vi "ClientProcess.vi"(0 "occurrence":refnum<k4>, 1 "target address":string, 2 "TCP port":u16, 5 "error in (no error)":errorcluster) -> (19 "error out":errorcluster)   [LabVIEW 2017, in "G#RemoteProxy.lvclass"]
doc: "Client process for the remote link to the target server process."
uses:
  G#RemoteProxy.lvclass
  G#Object/utils/G#Object_Event.ctl
  G#Object/utils/G#Object_EventType.ctl
  G#Object/utils/G#Object_ObjectInfoType.ctl
  G#Object/utils/G#Object_CreateMethod.ctl
  G#Object/G#Object.lvclass
  G#DebugServer/utils/LocalProcessData.ctl
  G#DebugServer/utils/TCPCommand.ctl
  G#Object/utils/G#Object_ClassInfoType.ctl
  G#Object/utils/G#Object_ClassHierarchy.ctl
  G#Debugger.lvlib
  G#DebugServer/G#DebugServer.lvclass
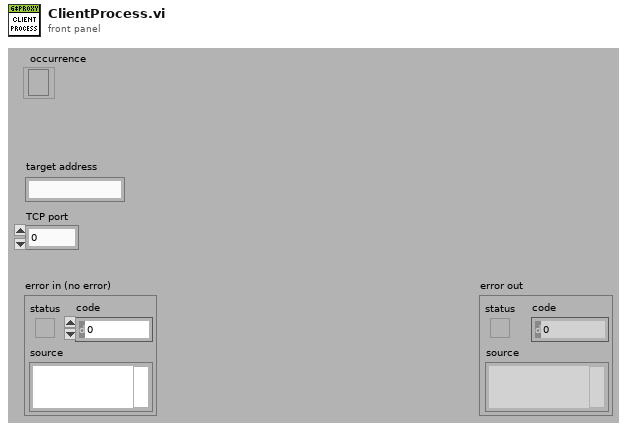
[diagram p1: front panel]
types:
  T1 = cluster{"connection ID":refnum<k5>, "Connected":bool}
  T2 = cluster{"connection ID":refnum<k5>, "Address":u32}
  T3 = typedef "G#Object.lvclass/G#Object_ClassInfoType.ctl" = cluster{"ClassName":string, "ObjectInfo":T4[], "ObjectRefs":refnum<class "G#Object.lvclass">[], "TypeRef":refnum<class "G#Object.lvclass">}
  T4 = typedef "G#Object.lvclass/G#Object_ObjectInfoType.ctl" = cluster{"ObjectName":string, "ObjectID":u32, "Users":i32, "Counter":bool, "AttributeRefs":u32[], "FullClassName":string, "ClassName":string, "CreateMethod":T5, "GenericDestructorExists":bool, "Owner":string}
  T5 = typedef "G#Object.lvclass/G#Object_CreateMethod.ctl" = enum16{"Create", "Create or look up existing", "Look up existing"}
  T6 = typedef "G#Object.lvclass/G#Object_ClassHierarchy.ctl" = cluster{"ClassName":string, "FullClassName":string, "ClassPath":path, "IsLeaf":bool}
  T7 = cluster{"AllObjects":T3, "class hierarchy":T6[]}[]
  T8 = typedef "G#DebugServer.lvclass/LocalProcessData.ctl" = cluster{"Event":string, "Command":T9, "Data":string, "Address":u32}
  T9 = typedef "G#DebugServer.lvclass/TCPCommand.ctl" = u8
  T10 = typedef "G#Object.lvclass/G#Object_Event.ctl" = cluster{"EventType":T11, "ObjectInfo":T4, "Ref":refnum<class "G#Object.lvclass">, "Time Stamp":timestamp, "LogText":string, "Parameters":variant[]}
  T11 = typedef "G#Object.lvclass/G#Object_EventType.ctl" = enum16{"Created new", "Looked up existing", "Deleted", "Forced delete", "Not deleted", "Garbage collected", "Cleared", "User", "Error", "External create object", "External create class attributes", "Created class attributes", "Run constructor", "Run constructor done", "Run open method", "Run open method done"}
  T12 = cluster{"G#DebugServerRef":refnum<class "G#Object.lvclass">, "attributes":variant[]}
  T13 = cluster{"G#DebugServerRef":refnum<class "G#Object.lvclass">, "ToString":string}
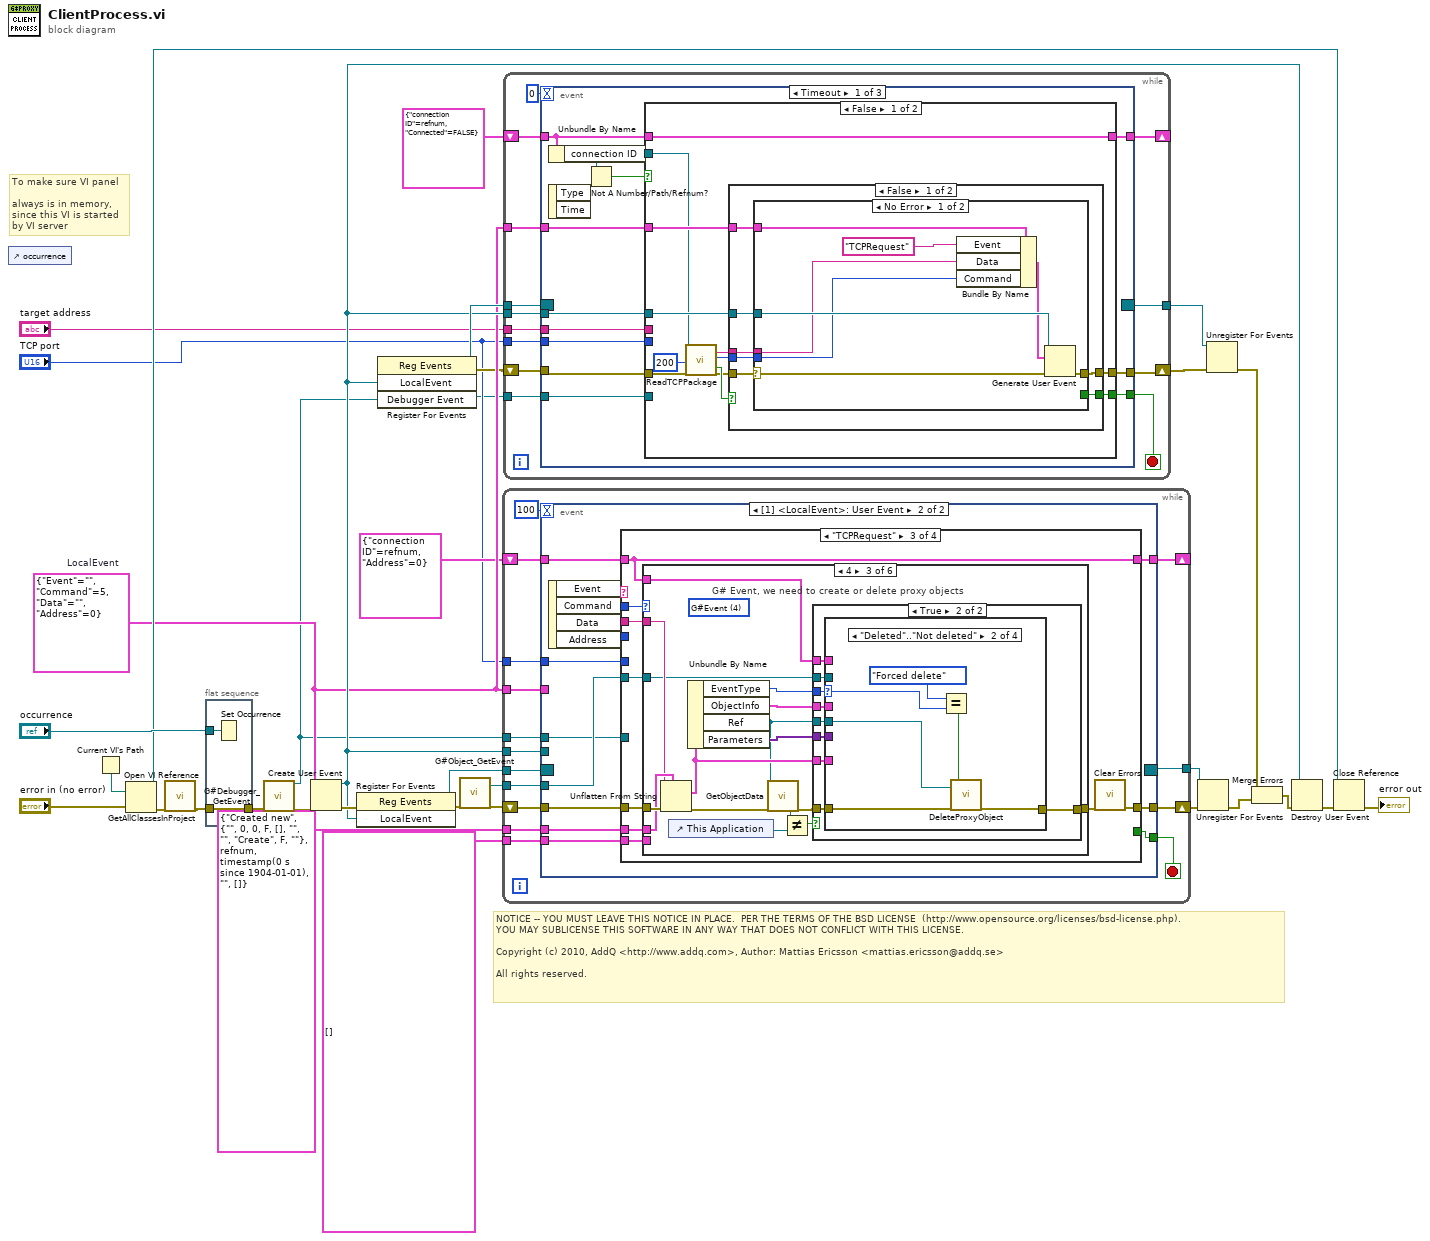
[diagram p0: block diagram]
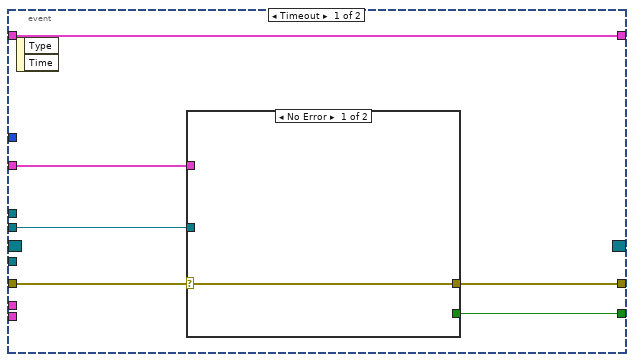
[diagram p2: hidden frame]
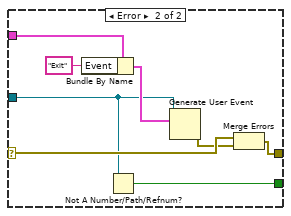
[diagram p3: hidden frame]
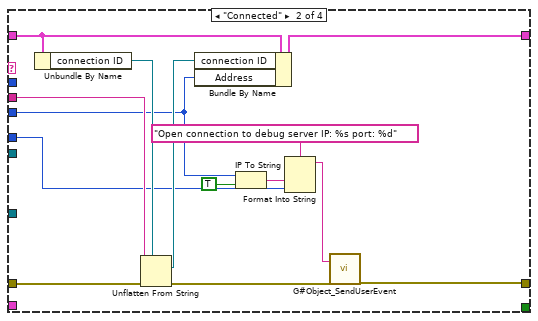
[diagram p5: hidden frame]
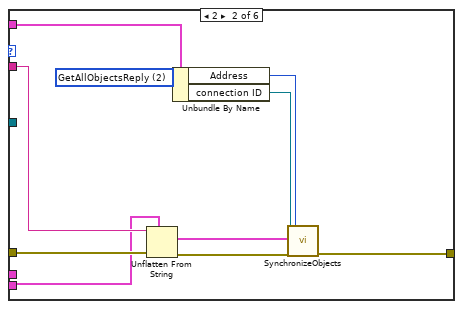
[diagram p7: hidden frame]
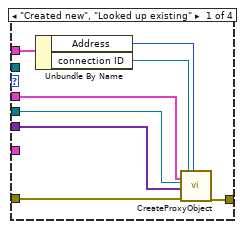
[diagram p9: hidden frame]
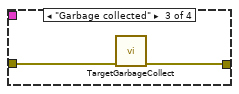
[diagram p10: hidden frame]
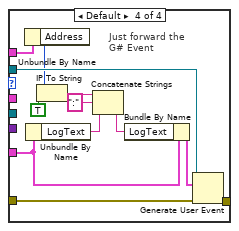
[diagram p11: hidden frame]
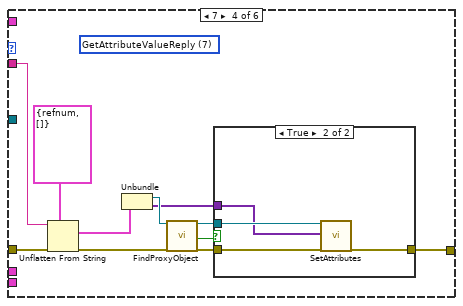
[diagram p12: hidden frame]
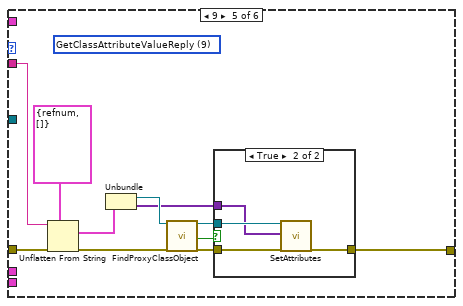
[diagram p14: hidden frame]
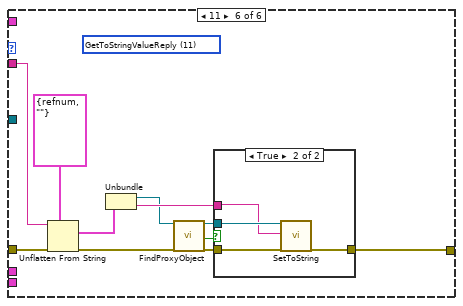
[diagram p16: hidden frame]
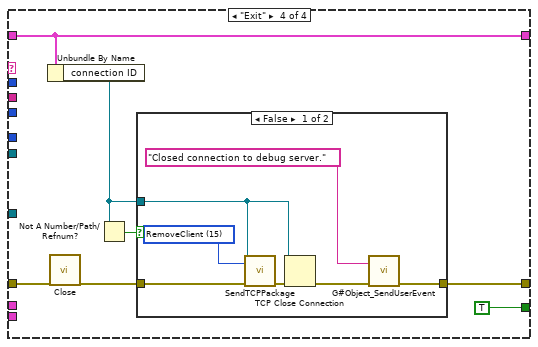
[diagram p18: hidden frame]
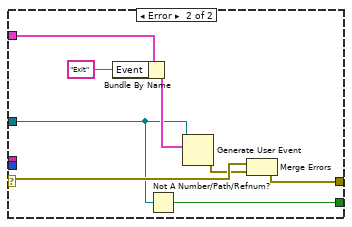
[diagram p20: hidden frame]
diagram:
  w12 = T8 {"Event"="", "Command"=5, "Data"="", "Address"=0}  # LocalEvent
  # "NOTICE -- YOU MUST LEAVE THIS NOTICE IN PLACE.  PER THE TERMS OF THE BSD LICENSE  (http://www.opensource.org/licenses/bsd-license.php).\nYOU MAY SUBLICENSE THIS SOFTWARE IN ANY WAY THAT DOES NOT CONFLICT WITH THIS LICENSE.\n\nCopyright (c) 2010, AddQ <http://www.addq.com>, Author: Mattias Ericsson <mattias.ericsson@addq.se>\n\nAll rights reserved."
  # "To make sure VI panel\n\nalways is in memory,\nsince this VI is started\nby VI server"
  n1 = control-ref of="occurrence"() -> ()  [unwired: 1 out]
  n2 = Current VI's Path() -> (path=w33:path)
  n3 = Open VI Reference(vi path=w33, error in (no error)="error in (no error)") -> (vi reference=w29:refnum<vi>, error out=w10:errorcluster)  [unwired: 4 in]
  n4 = call "GetAllClassesInProject.vi"("error in (no error)"=w10) -> ("error out"=w6:errorcluster)  [unwired: 15 in, 3 out]
  n5 = flat-sequence {
    tunnel: "occurrence" -> [w35]
    tunnel: w6 -> [w34]
    tunnel: [w34] -> w9
    frame #0 {
      n6 = Set Occurrence(w35) -> ()
    }
  }
  n7 = call "G#Debugger_GetEvent.vi"("error in (no error)"=w9) -> ("Debugger Event"=w2:refnum<user-event>, "error out"=w28:errorcluster)  [unwired: 17 in]
  n8 = Create User Event(user event datatype=w12, error in=w28) -> (user event=w13:refnum<user-event>, error out=w27:errorcluster)
  n9 = register-events(error in=w27, w13) -> (reference out=w19:refnum<event-registration>, error out=w26:errorcluster)  [unwired: 1 in]
  n10 = register-events(w13, w2) -> (reference out=w24:refnum<event-registration>, error out=w4:errorcluster)  [unwired: 2 in]
  n11 = call "G#Object_GetEvent.vi"("error in (no error)"=w26) -> ("G# event"=w15:refnum<user-event>, "error out"=w25:errorcluster)  [unwired: 14 in, 3 out]
  n12 = while {
    shift-right: [w46] -> w21
    shift-left: w25 -> [w49]
    tunnel: [w50] -> w20
    tunnel: w19 -> [w48]
    tunnel: w13 -> [w45]
    tunnel: w15 -> [w43]
    tunnel: T10 {"EventType"=enum."Created new", "ObjectInfo"={"ObjectName"="", "ObjectID"=0, "Users"=0, "Counter"=FALSE, "AttributeRefs"=[], "FullClassName"="", "ClassName"="", "CreateMethod"=enum."Create", "GenericDestructorExists"=FALSE, "Owner"=""}, "Ref"=refnum, "Time Stamp"=timestamp(0 s since 1904-01-01), "LogText"="", "Parameters"=[]} ("event data") -> [w42]
    tunnel: w12 -> [w41]
    tunnel: T7 [] ("TargetClassInfo") -> [w40]
    shift-right: [w38] -> _
    shift-left: T2 {"connection ID"=refnum, "Address"=0} -> [w39]
    tunnel: "TCP port" -> [w37]
    tunnel: w2 -> [w36]
    stop <- w44 stop-if-true
    n13 = event shown="[1] <LocalEvent>: User Event" {
      selector: w48 -> [_ _]
      dyn-events: [_ _] -> w50
      timeout: 100 -> [_ _]
      tunnel: w49 -> [w56 w78]
      tunnel: [w54 w77] -> w46
      tunnel: w45 -> [w55 _]
      tunnel: [w52 w76] -> w44
      tunnel: w43 -> [_ w73]
      tunnel: w42 -> [_ w72]
      tunnel: w41 -> [w53 _]
      tunnel: w40 -> [_ w71]
      tunnel: w39 -> [w51 w70]
      tunnel: [w51 w69] -> w38
      tunnel: w37 -> [_ w67]
      tunnel: w36 -> [_ w66]
      event Timeout {
        n14 = event-data() -> ()  [unwired: 1 in, 2 out]
        n15 = case shown="No Error" w56 {
          selector: w56 -> [w57 w64]
          tunnel: w55 -> [_ w59]
          tunnel: [w57 w65] -> w54
          tunnel: w53 -> [_ w62]
          tunnel: [_ w58] -> w52
          frame No Error {
          }
          frame Error {
            n16 = Bundle By Name(cluster=w62, "Event"="Exit") -> (w61:T8)
            n17 = Not A Number/Path/Refnum?(number/path/refnum=w59) -> (NaN/Path/Refnum?=w58:bool)
            n18 = Generate User Event(user event=w59, event data cluster=w61) -> (error out=w63:errorcluster)  [unwired: 2 in, 1 out]
            n19 = Merge Errors(w64, w63) -> (w65:errorcluster)
          }
        }
      }
      event User Event {
        n20 = event-data() -> ("Event"=w79:string, "Command"=w75:T9, "Data"=w74:string, "Address"=w68:u32)  [unwired: 1 in]
        n21 = case shown="\"TCPRequest\"" w79 {
          tunnel: w78 -> [w81 w95 w101 w222]
          tunnel: [w81 w82 w97 w219] -> w77
          tunnel: [_ _ _ TRUE] -> w76
          tunnel: w75 -> [_ _ w104 _]
          tunnel: w74 -> [_ w94 w103 _]
          tunnel: w73 -> [_ _ w102 _]
          tunnel: w72 -> [_ _ w100 _]
          tunnel: w71 -> [_ _ w99 _]
          tunnel: w70 -> [w80 w92 w96 w218]
          tunnel: [w80 w91 w96 w218] -> w69
          tunnel: w68 -> [_ w85 _ _]
          tunnel: w67 -> [_ w83 _ _]
          tunnel: w66 -> [_ _ _ _]
          frame Default {
          }
          frame "Connected" {
            n22 = Unbundle By Name(w92) -> ("connection ID"=w93:refnum<k5>)
            n23 = Unflatten From String(type=w93, binary string=w94, error in (no error)=w95) -> (value=w90:refnum<k5>, error out=w89:errorcluster)  [unwired: 2 in, 1 out]
            n24 = Bundle By Name(cluster=w92, "connection ID"=w90, "Address"=w85) -> (w91:T2)
            n25 = IP To String(1:TRUE ("dot notation? (F)"), 2:w85) -> (0:w86:string)
            n26 = Format Into String(format string="Open connection to debug server IP: %s port: %d", w86, w83) -> (resulting string=w87:string)  [unwired: 2 in, 1 out]
            n27 = call "G#Object_SendUserEvent.vi"("text"=w87, "error in (no error)"=w89) -> ("error out"=w82:errorcluster)  [unwired: 16 in, 1 out]
          }
          frame "TCPRequest" {
            n28 = case shown="4" w104 {
              tunnel: w103 -> [_ w113 w128 w178 w194 w210]
              tunnel: w102 -> [_ _ w124 _ _ _]
              tunnel: w101 -> [w105 w114 w130 w179 w195 w211]
              tunnel: [w105 w109 w126 w175 w185 w206] -> w98
              tunnel: w100 -> [_ _ w129 _ _ _]
              tunnel: w99 -> [_ w112 _ _ _ _]
              tunnel: w96 -> [_ w108 w115 _ _ _]
              frame Default {
              }
              frame 2 {
                (unwired) T9 2 items=["GarbageCollect", "GetAllObjects", "GetAllObjectsReply", "CleanUp", "G#Event"] ("Command")
                n29 = Unflatten From String(type=w112, binary string=w113, error in (no error)=w114) -> (value=w110:T7, error out=w111:errorcluster)  [unwired: 2 in, 1 out]
                n30 = Unbundle By Name(w108) -> ("Address"=w107:u32, "connection ID"=w106:refnum<k5>)
                n31 = call "SynchronizeObjects.vi"("connection ID"=w106, "TargetClassInfo"=w110, "error in (no error)"=w111, "address"=w107) -> ("error out"=w109:errorcluster)  [unwired: 15 in]
              }
              frame 4 {
                (unwired) T9 4 items=["GarbageCollect", "GetAllObjects", "GetAllObjectsReply", "CleanUp", "G#Event"] ("Command")
                # "G# Event, we need to create or delete proxy objects"
                n32 = Unflatten From String(type=w129, binary string=w128, error in (no error)=w130) -> (value=w123:T10, error out=w120:errorcluster)  [unwired: 2 in, 1 out]
                n33 = control-ref of="This Application"() -> (w116:refnum<vi>)
                n34 = Unbundle By Name(w123) -> ("EventType"=w127:T11, "ObjectInfo"=w125:T4, "Ref"=w119:refnum<class "G#Object.lvclass">, "Parameters"=w122:variant[])
                n35 = call "GetObjectData.vi"("remote ref"=w119, "error in (no error)"=w120) -> ("AppRefnum"=w117:refnum<vi>, "error out"=w121:errorcluster)  [unwired: 13 in, 3 out]
                n36 = Not Equal?(x=w117, y=w116) -> (x != y?=w118:bool)
                n37 = case shown="True" w118 {
                  tunnel: w127 -> [_ w140]
                  tunnel: w121 -> [w131 w139]
                  tunnel: [w131 w138] -> w126
                  tunnel: w125 -> [_ w137]
                  tunnel: w119 -> [_ w136]
                  tunnel: w124 -> [_ w135]
                  tunnel: w123 -> [_ w134]
                  tunnel: w122 -> [_ w133]
                  tunnel: w115 -> [_ w132]
                  frame False {
                    # "Debug server is running on the\nsame application instance as the debugger,\nthe debugger will catch the event by him self!"
                  }
                  frame True {
                    n38 = case shown="\"Deleted\"..\"Not deleted\"" w140 {
                      selector: w140 -> [_ w151 _ _]
                      tunnel: w139 -> [w148 w154 w156 w168]
                      tunnel: [w147 w153 w155 w167] -> w138
                      tunnel: w137 -> [w144 _ _ _]
                      tunnel: w136 -> [w146 w152 _ _]
                      tunnel: w135 -> [_ _ _ w166]
                      tunnel: w134 -> [_ _ _ w165]
                      tunnel: w133 -> [w145 _ _ _]
                      tunnel: w132 -> [w143 _ _ w160]
                      frame "Created new", "Looked up existing" {
                        n39 = Unbundle By Name(w143) -> ("Address"=w142:u32, "connection ID"=w141:refnum<k5>)
                        n40 = call "CreateProxyObject.vi"("object info"=w144, "remote object ref"=w146, "parameters"=w145, "error in (no error)"=w148, "connection ID"=w141, "address"=w142) -> ("error out"=w147:errorcluster)  [unwired: 13 in]
                      }
                      frame "Deleted".."Not deleted" {
                        n41 = Equal?(x=G#Object_EventType."Forced delete" ("EventType"), y=w151) -> (x = y?=w149:bool)
                        n42 = call "DeleteProxyObject.vi"("remote object ref"=w152, "error in (no error)"=w154, "force delete? (F)"=w149) -> ("error out"=w153:errorcluster)  [unwired: 16 in]
                      }
                      frame "Garbage collected" {
                        n43 = call "TargetGarbageCollect.vi"("error in (no error)"=w156) -> ("error out"=w155:errorcluster)  [unwired: 18 in]
                      }
                      frame Default {
                        # "Just forward the\nG# Event"
                        n44 = Unbundle By Name(w160) -> ("Address"=w158:u32)
                        n45 = Unbundle By Name(w165) -> ("LogText"=w163:string)
                        n46 = IP To String(1:TRUE ("dot notation? (F)"), 2:w158) -> (0:w159:string)
                        n47 = Concatenate Strings(w159, ":" ("string"), w163) -> (w162:string)
                        n48 = Bundle By Name(cluster=w165, "LogText"=w162) -> (w164:T10)
                        n49 = Generate User Event(user event=w166, event data cluster=w164, error in=w168) -> (error out=w167:errorcluster)  [unwired: 1 in, 1 out]
                      }
                    }
                  }
                }
              }
              frame 7 {
                (unwired) T9 7 items=["GarbageCollect", "GetAllObjects", "GetAllObjectsReply", "CleanUp", "G#Event", "RegisterClient", "GetAttributeValue", "GetAttributeValueReply", "GetClassAttributeValue", "GetClassAttributeValueReply", "GetToStringValue", "GetToStringValueReply", "GetClassHierarchy", "GetClassHierarchyReply"] ("Command")
                n50 = Unflatten From String(type=T12 {"G#DebugServerRef"=refnum, "attributes"=[]} ("cluster"), binary string=w178, error in (no error)=w179) -> (value=w176:T12, error out=w174:errorcluster)  [unwired: 2 in, 1 out]
                n51 = Unbundle(w176) -> ("G#DebugServerRef"=w172:refnum<class "G#Object.lvclass">, "attributes"=w169:variant[])
                n52 = call "FindProxyObject.vi"("remote ref"=w172, "error in (no error)"=w174) -> ("proxy ref"=w171:refnum<class "G#RemoteProxy.lvclass">, "found"=w170:bool, "error out"=w173:errorcluster)  [unwired: 15 in]
                n53 = case shown="True" w170 {
                  tunnel: w173 -> [w180 w182]
                  tunnel: [w180 w184] -> w175
                  tunnel: w171 -> [_ w183]
                  tunnel: w169 -> [_ w181]
                  frame False {
                  }
                  frame True {
                    n54 = call "SetAttributes.vi"("reference in"=w183, "attributes"=w181, "error in (no error)"=w182) -> ("error out"=w184:errorcluster)  [unwired: 15 in, 1 out]
                  }
                }
              }
              frame 9 {
                (unwired) T9 9 items=["GarbageCollect", "GetAllObjects", "GetAllObjectsReply", "CleanUp", "G#Event", "RegisterClient", "GetAttributeValue", "GetAttributeValueReply", "GetClassAttributeValue", "GetClassAttributeValueReply", "GetToStringValue", "GetToStringValueReply", "GetClassHierarchy", "GetClassHierarchyReply"] ("Command")
                n55 = Unflatten From String(type=T12 {"G#DebugServerRef"=refnum, "attributes"=[]} ("cluster"), binary string=w194, error in (no error)=w195) -> (value=w192:T12, error out=w191:errorcluster)  [unwired: 2 in, 1 out]
                n56 = Unbundle(w192) -> ("G#DebugServerRef"=w189:refnum<class "G#Object.lvclass">, "attributes"=w186:variant[])
                n57 = call "FindProxyClassObject.vi"("remote class ref"=w189, "error in (no error)"=w191) -> ("proxy class ref"=w188:refnum<class "G#RemoteProxy.lvclass">, "found"=w187:bool, "error out"=w190:errorcluster)  [unwired: 15 in]
                n58 = case shown="True" w187 {
                  tunnel: w190 -> [w196 w200]
                  tunnel: [w196 w199] -> w185
                  tunnel: w188 -> [_ w198]
                  tunnel: w186 -> [_ w197]
                  frame False {
                  }
                  frame True {
                    n59 = call "SetAttributes.vi"("reference in"=w198, "attributes"=w197, "error in (no error)"=w200) -> ("error out"=w199:errorcluster)  [unwired: 15 in, 1 out]
                  }
                }
              }
              frame 11 {
                (unwired) T9 11 items=["GarbageCollect", "GetAllObjects", "GetAllObjectsReply", "CleanUp", "G#Event", "RegisterClient", "GetAttributeValue", "GetAttributeValueReply", "GetClassAttributeValue", "GetClassAttributeValueReply", "GetToStringValue", "GetToStringValueReply", "GetClassHierarchy", "GetClassHierarchyReply"] ("Command")
                n60 = Unflatten From String(type=T13 {"G#DebugServerRef"=refnum, "ToString"=""} ("cluster"), binary string=w210, error in (no error)=w211) -> (value=w208:T13, error out=w205:errorcluster)  [unwired: 2 in, 1 out]
                n61 = Unbundle(w208) -> ("G#DebugServerRef"=w201:refnum<class "G#Object.lvclass">, "ToString"=w207:string)
                n62 = call "FindProxyObject.vi"("remote ref"=w201, "error in (no error)"=w205) -> ("proxy ref"=w202:refnum<class "G#RemoteProxy.lvclass">, "found"=w203:bool, "error out"=w204:errorcluster)  [unwired: 15 in]
                n63 = case shown="True" w203 {
                  tunnel: w204 -> [w212 w216]
                  tunnel: [w212 w215] -> w206
                  tunnel: w202 -> [_ w214]
                  tunnel: w207 -> [_ w213]
                  frame False {
                  }
                  frame True {
                    n64 = call "SetToString.vi"("reference in"=w214, "to string"=w213, "error in (no error)"=w216) -> ("error out"=w215:errorcluster)  [unwired: 15 in, 1 out]
                  }
                }
              }
            }
            n65 = call <vilib>:"Clear Errors.vi"("error in (no error)"=w98) -> ("error out"=w97:errorcluster)  [unwired: 5 in, 1 out]
          }
          frame "Exit" {
            n66 = Unbundle By Name(w218) -> ("connection ID"=w217:refnum<k5>)
            n67 = call "Close.vi"("error in (no error)"=w222) -> ("error out"=w221:errorcluster)  [unwired: 18 in]
            n68 = Not A Number/Path/Refnum?(number/path/refnum=w217) -> (NaN/Path/Refnum?=w220:bool)
            n69 = case shown="False" w220 {
              tunnel: w221 -> [w230 w231]
              tunnel: w217 -> [w228 _]
              tunnel: [w225 w231] -> w219
              frame False {
                w227 = T9 15 items=["GarbageCollect", "GetAllObjects", "GetAllObjectsReply", "CleanUp", "G#Event", "RegisterClient", "GetAttributeValue", "GetAttributeValueReply", "GetClassAttributeValue", "GetClassAttributeValueReply", "GetToStringValue", "GetToStringValueReply", "GetClassHierarchy", "GetClassHierarchyReply", "Destroy", "RemoveClient"] ("Command")
                n70 = call "SendTCPPackage.vi"("connection ID"=w228, "command"=w227, "error in (no error)"=w230) -> ("error out"=w229:errorcluster)  [unwired: 16 in]
                n71 = TCP Close Connection(connection ID=w228, error in (no error)=w229) -> (error out=w226:errorcluster)  [unwired: 1 in, 1 out]
                n72 = call "G#Object_SendUserEvent.vi"("text"="Closed connection to debug server.", "error in (no error)"=w226) -> ("error out"=w225:errorcluster)  [unwired: 16 in, 1 out]
              }
              frame True {
              }
            }
          }
        }
      }
    }
  }
  n73 = while {
    shift-right: [w240] -> w23
    shift-left: w4 -> [w241]
    tunnel: w24 -> [w244]
    tunnel: [w243] -> w22
    tunnel: w13 -> [w238]
    tunnel: w12 -> [w237]
    shift-right: [w235] -> _
    shift-left: T1 {"connection ID"=refnum, "Connected"=FALSE} -> [w234]
    tunnel: "target address" -> [w236]
    tunnel: "TCP port" -> [w233]
    tunnel: w2 -> [w232]
    stop <- w239 stop-if-true
    n74 = event shown="[0] Timeout" {
      selector: w244 -> [_ _ _]
      dyn-events: [_ _ _] -> w243
      timeout: 0 -> [_ _ _]
      tunnel: w241 -> [w255 w348 w365]
      tunnel: [w256 w350 w364] -> w240
      tunnel: [w252 w347 _] -> w239
      tunnel: w238 -> [w254 _ w366]
      tunnel: w237 -> [w253 _ _]
      tunnel: w236 -> [w251 _ _]
      tunnel: [w250 w345 w362] -> w235
      tunnel: w234 -> [w246 w345 w362]
      tunnel: w233 -> [w248 _ _]
      tunnel: w232 -> [w247 _ _]
      event Timeout {
        n75 = Unbundle By Name(w246) -> ("connection ID"=w245:refnum<k5>)
        n76 = event-data() -> ()  [unwired: 1 in, 2 out]
        n77 = Not A Number/Path/Refnum?(number/path/refnum=w245) -> (NaN/Path/Refnum?=w249:bool)
        n78 = case shown="False" w249 {
          tunnel: [w267 w298] -> w256
          tunnel: w255 -> [w266 w304]
          tunnel: w254 -> [w264 w301]
          tunnel: w253 -> [w260 _]
          tunnel: [w259 w299] -> w252
          tunnel: w251 -> [_ w300]
          tunnel: [w257 w293] -> w250
          tunnel: w246 -> [w257 w294]
          tunnel: w248 -> [_ w297]
          tunnel: w247 -> [_ w296]
          tunnel: w245 -> [w258 _]
          frame False {
            n79 = call "ReadTCPPackage.vi"("connection ID"=w258, "timeout ms (200)"=200 ("timeout ms (25000)"), "error in (no error)"=w266) -> ("payload"=w263:string, "command"=w262:T9, "timeout"=w268:bool, "error out"=w265:errorcluster)  [unwired: 13 in]
            n80 = case shown="False" w268 {
              tunnel: w265 -> [w275 w292]
              tunnel: [w273 w292] -> w267
              tunnel: w264 -> [w274 _]
              tunnel: w260 -> [w272 _]
              tunnel: w263 -> [w271 _]
              tunnel: w262 -> [w270 _]
              tunnel: [w269 _] -> w259
              frame False {
                n81 = case shown="No Error" w275 {
                  selector: w275 -> [w278 w290]
                  tunnel: w274 -> [w283 w285]
                  tunnel: [w282 w291] -> w273
                  tunnel: w272 -> [w281 w288]
                  tunnel: w271 -> [w277 _]
                  tunnel: w270 -> [w276 _]
                  tunnel: [_ w284] -> w269
                  frame No Error {
                    n82 = Bundle By Name(cluster=w281, "Event"="TCPRequest" ("Command"), "Data"=w277, "Command"=w276) -> (w280:T8)
                    n83 = Generate User Event(user event=w283, event data cluster=w280, error in=w278) -> (error out=w282:errorcluster)  [unwired: 1 in, 1 out]
                  }
                  frame Error {
                    n84 = Bundle By Name(cluster=w288, "Event"="Exit" ("Command")) -> (w287:T8)
                    n85 = Not A Number/Path/Refnum?(number/path/refnum=w285) -> (NaN/Path/Refnum?=w284:bool)
                    n86 = Generate User Event(user event=w285, event data cluster=w287) -> (error out=w289:errorcluster)  [unwired: 2 in, 1 out]
                    n87 = Merge Errors(w290, w289) -> (w291:errorcluster)
                  }
                }
              }
              frame True {
                # "TCP timeout"
              }
            }
          }
          frame True {
            n88 = TCP Open Connection(address=w300, remote port or service name=w297, timeout ms (60000)=200, error in (no error)=w304) -> (connection ID=w295:refnum<k5>, error out=w302:errorcluster)  [unwired: 1 in]
            n89 = case shown="No Error" w302 {
              selector: w302 -> [w321 w339]
              tunnel: [w310 w336] -> w298
              tunnel: w301 -> [w326 w338]
              tunnel: [_ w334] -> w299
              tunnel: w300 -> [w322 _]
              tunnel: w295 -> [w307 _]
              tunnel: w296 -> [w309 w333]
              tunnel: w294 -> [w308 w332]
              tunnel: [w306 w327] -> w293
              frame No Error {
                w316 = T8 {"Event"="TCPCommand", "Command"=5, "Data"="", "Address"=0}  # LocalData
                w325 = T8 {"Event"="Connected", "Command"=0, "Data"="", "Address"=0}  # LocalData
                n90 = Flatten To String(anything=w307, error in (no error)=w321) -> (data string=w319:string, error out=w320:errorcluster)  [unwired: 2 in, 1 out]
                n91 = String To IP(1:w322) -> (0:w323:u32)
                n92 = Bundle By Name(cluster=w308, "Connected"=TRUE, "connection ID"=w307) -> (w306:T1)
                n93 = Bundle By Name(cluster=w325, "Address"=w323, "Data"=w319) -> (w324:T8)
                n94 = Generate User Event(user event=w326, event data cluster=w324, error in=w320) -> (user event out=w317:refnum<user-event>, error out=w318:errorcluster)  [unwired: 1 in]
                n95 = Generate User Event(user event=w317, event data cluster=w316, error in=w318) -> (user event out=w315:refnum<user-event>, error out=w314:errorcluster)  [unwired: 1 in]
                n96 = Generate User Event(user event=w315, event data cluster=T8 {"Event"="TCPCommand", "Command"=1, "Data"="", "Address"=0} ("event data"), error in=w314) -> (error out=w311:errorcluster)  [unwired: 1 in, 1 out]
                n97 = Generate User Event(user event=w309, event data cluster="Connected" ("event data"), error in=w311) -> (error out=w310:errorcluster)  [unwired: 1 in, 1 out]
              }
              frame Error {
                n98 = Unbundle By Name(w332) -> ("Connected"=w331:bool)
                n99 = call <vilib>:"Clear Errors.vi"("error in (no error)"=w339) -> ("error out"=w337:errorcluster)  [unwired: 5 in, 1 out]
                n100 = Not A Number/Path/Refnum?(number/path/refnum=w338) -> (NaN/Path/Refnum?=w335:bool)
                n101 = Not A Number/Path/Refnum?(number/path/refnum=w333) -> (NaN/Path/Refnum?=w330:bool)
                n102 = Compound Arithmetic op=AND(w331, invert w330) -> (w329:bool)
                n103 = case shown="True" w329 {
                  tunnel: w337 -> [w340 w344]
                  tunnel: [w340 w343] -> w336
                  tunnel: w333 -> [_ w342]
                  frame False {
                  }
                  frame True {
                    n104 = Generate User Event(user event=w342, event data cluster="Disconnected" ("event data"), error in=w344) -> (error out=w343:errorcluster)  [unwired: 1 in, 1 out]
                  }
                }
                n105 = Bundle By Name(cluster=w332, "Connected"=FALSE) -> (w327:T1)
                n106 = Or(x=w335, y=w330) -> (x .or. y?=w334:bool)
              }
            }
          }
        }
      }
      event User Event {
        n107 = event-data() -> ("Event"=w349:string, "Command"=w346:T9)  [unwired: 1 in, 5 out]
        n108 = case shown="\"TCPCommand\"" w349 {
          tunnel: w348 -> [w351 w356 w361]
          tunnel: [w351 w359 w361] -> w350
          tunnel: [_ _ TRUE] -> w347
          tunnel: w346 -> [_ w358 _]
          tunnel: w345 -> [_ w353 _]
          frame Default {
          }
          frame "TCPCommand" {
            n109 = Unbundle By Name(w353) -> ("connection ID"=w352:refnum<k5>)
            n110 = control-ref of="This Application"() -> (w357:refnum<vi>)
            n111 = Flatten To String(anything=w357, error in (no error)=w356) -> (data string=w354:string, error out=w355:errorcluster)  [unwired: 2 in, 1 out]
            n112 = call "SendTCPPackage.vi"("connection ID"=w352, "command"=w358, "data"=w354, "error in (no error)"=w355) -> ("error out"=w359:errorcluster)  [unwired: 15 in]
          }
          frame "Exit" {
          }
        }
      }
      event User Event {
        n113 = event-data() -> ("GUI event"=w363:string)  [unwired: 1 in, 3 out]
        n114 = case shown="\"Refresh\"" w363 {
          tunnel: w365 -> [w367 w368 w375 w379 w383]
          tunnel: [w367 w369 w372 w376 w382] -> w364
          tunnel: w366 -> [_ w371 w374 w377 w381]
          frame Default {
          }
          frame "Refresh" {
            n115 = Generate User Event(user event=w371, event data cluster=T8 {"Event"="TCPCommand", "Command"=1, "Data"="", "Address"=0} ("event data"), error in=w368) -> (error out=w369:errorcluster)  [unwired: 1 in, 1 out]
          }
          frame "Clear" {
            n116 = Generate User Event(user event=w374, event data cluster=T8 {"Event"="TCPCommand", "Command"=0, "Data"="", "Address"=0} ("event data"), error in=w375) -> (error out=w372:errorcluster)  [unwired: 1 in, 1 out]
          }
          frame "Clear object tab" {
            n117 = Generate User Event(user event=w377, event data cluster=T8 {"Event"="TCPCommand", "Command"=3, "Data"="", "Address"=0} ("event data"), error in=w379) -> (error out=w376:errorcluster)  [unwired: 1 in, 1 out]
          }
          frame "Exit", "Stop" {
            # "Tell other loop to quit"
            # "Debugger is closing -> Exit"
            n118 = Generate User Event(user event=w381, event data cluster=T8 {"Event"="Exit", "Command"=0, "Data"="", "Address"=0} ("event data"), error in=w383) -> (error out=w382:errorcluster)  [unwired: 1 in, 1 out]
          }
        }
      }
    }
  }
  n119 = Unregister For Events(event registration refnum=w20, error in=w21) -> (error out=w17:errorcluster)
  n120 = Unregister For Events(event registration refnum=w22, error in=w23) -> (error out=w18:errorcluster)
  n121 = Merge Errors(w18, w17) -> (w16:errorcluster)
  n122 = Destroy User Event(user event=w13, error in=w16) -> (error out=w8:errorcluster)
  n123 = Close Reference(reference=w29, error in (no error)=w8) -> (error out=→"error out":errorcluster)
